vi "XYZ.vi"() -> ()   [LabVIEW 2023]
uses:
  <vilib>/Utility/miscctls.llb/LV3DPointTypeDef.ctl
  <vilib>/picture/3D Picture Control/Object/Create Object (drawable).vi
  <vilib>/picture/3D Picture Control/Object/Add Object (no reference).vi
  <vilib>/picture/3D Picture Control/NI_3D Picture Control.lvlib
panel:
  in  "Up Direction":T1
  in  "Target":T1
  in  "Camera Position":T1
  in  "stop":bool
  in  "Axis label?":bool
  in  "Half plane?":bool=TRUE
  out "3D Picture":refnum<vi>(3d-picture)
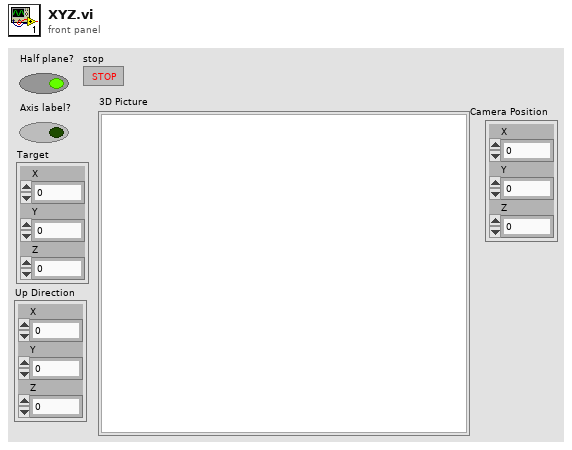
[diagram p1: front panel]
types:
  T1 = typedef "LV3DPointTypeDef.ctl" = cluster{"X":sgl, "Y":sgl, "Z":sgl}
  T2 = cluster{"Red":sgl, "Green":sgl, "Blue":sgl, "Alpha":sgl}
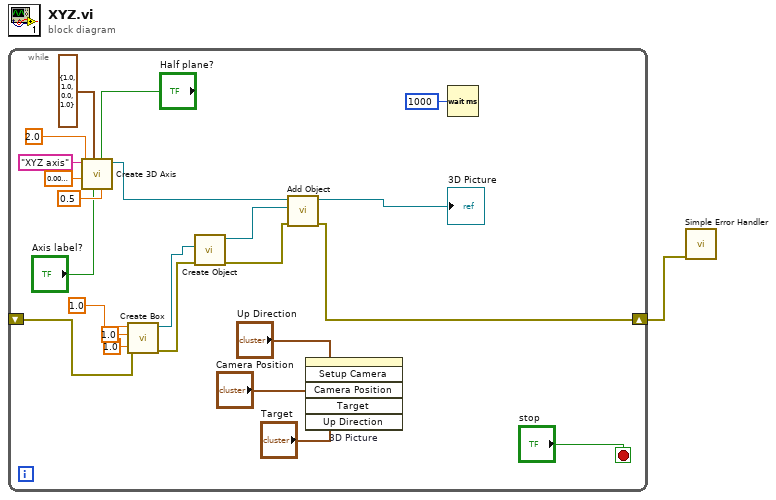
[diagram p0: block diagram]
diagram:
  n1 = while {
    shift-right: [w9] -> w1
    shift-left: _ -> [w8]
    stop <- "stop" stop-if-true
    n2 = call <vilib>:"Create 3D Axis.vi"("Character Size"=sgl 0.5, "Half plane?"="Half plane?", "Axis label?"="Axis label?", "Color"=T2 {"Red"=1.0, "Green"=1.0, "Blue"=0.0, "Alpha"=1.0}, "Radius"=sgl 0.01, "Length"=sgl 2.0, "Name"="XYZ axis") -> ("New Object Refnum"=w23:refnum<vi>)  [unwired: 3 in, 1 out]
    n3 = call <vilib>:"Create Box.vi"("error in (no error)"=w8, "Length Z"=sgl 1.0, "Length Y"=sgl 1.0, "Length X"=sgl 1.0) -> ("error out"=w11:errorcluster, "New Box Refnum"=w15:refnum<vi>)  [unwired: 6 in]
    n4 = call-poly <vilib>:"Create Object.vi"("error in (no error)"=w11, "Geometry"=w15) -> ("error out"=w10:errorcluster, "Scene:New Object"=w22:refnum<vi>)  [unwired: 8 in]
    n5 = call-poly <vilib>:"Add Object.vi"("error in (no error)"=w10, "New Object In"=w22, "Scene Object In"=w23) -> ("error out"=w9:errorcluster, "Scene Object Out"=→"3D Picture":refnum<vi>)  [unwired: 7 in]
    n6 = invoke on="3D Picture" class="SceneGraphDisp (strict)" method="Setup Camera"("Camera Position"="Camera Position", "Target"="Target", "Up Direction"="Up Direction") -> ()  [unwired: 3 in, 6 out]
    n7 = Wait (ms)(milliseconds to wait=u32 1000) -> ()  [unwired: 1 out]
  }
  n8 = call <vilib>:"Simple Error Handler.vi"("error in (no error)"=w1) -> ()  [unwired: 4 in, 5 out]
